vi "Close PG.vi"(8 "error in (no error)":errorcluster, 11 "Data.PG in":refnum<class "Data.PGSQL.lvclass">) -> (0 "error out":errorcluster, 3 "Data.PG out":refnum<class "Data.PGSQL.lvclass">)   [LabVIEW 2013, in "Data.PGSQL.lvclass"]
uses:
  Data.PGSQL.lvclass
  PostgreSQL Library/Connection/PQ Connection.lvclass
  Data.PGSQL.lvclass/Data.PGSQL.ctl
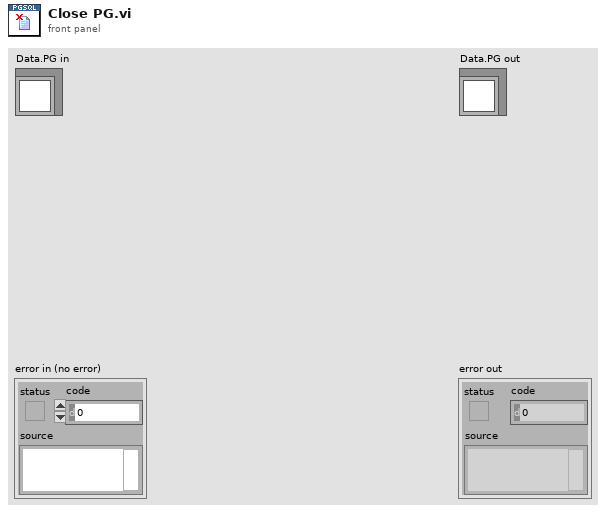
[diagram p1: front panel]
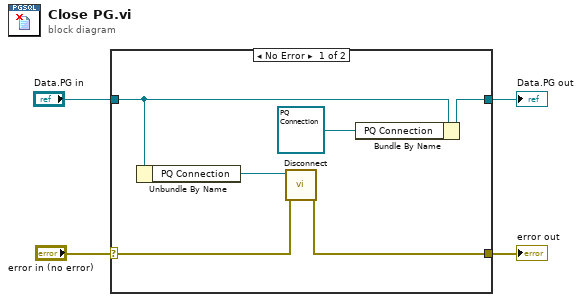
[diagram p0: block diagram]
diagram:
  n1 = case shown="No Error" "error in (no error)" {
    selector: "error in (no error)" -> [w8 w12]
    tunnel: [w9 w11] -> w4
    tunnel: "Data.PG in" -> [w6 w11]
    tunnel: [w7 w12] -> w1
    frame No Error {
      n2 = Unbundle By Name(w6) -> ("PQ Connection"=w5:refnum<class "PQ Connection.lvclass">)
      n3 = call-dynamic "Disconnect.vi"("error in (no error)"=w8, "PQ Connection in"=w5) -> ("error out"=w7:errorcluster)  [unwired: 9 in]
      n4 = Bundle By Name(cluster=w6, "PQ Connection"=refnum<class "PQ Connection.lvclass"> refnum) -> (w9:refnum<class "Data.PGSQL.lvclass">)
    }
    frame Error {
    }
  }
  "error out" <- w1
  "Data.PG out" <- w4
